vi "Default or Users Font.vi"(0 "PDF Report":refnum<class "PDF Report Class.lvclass">, 5 "Font":T1={"Name"="", "Size"=-1.0, "Color"=0, "Style"={"Bold"=FALSE, "Italic"=FALSE, "Underline"=FALSE, "Strikeout"=FALSE}, "Type"={"Type&direction"=enum."Select", "Embedded"=FALSE, "Encoding"=""}}, 11 "error in (no error)":errorcluster) -> (4 "PDF Report duplicate":refnum<class "PDF Report Class.lvclass">, 6 "Font OUT":T1={"Name"="Helvetica", "Size"=12.0, "Color"=0, "Style"={"Bold"=FALSE, "Italic"=FALSE, "Underline"=FALSE, "Strikeout"=FALSE}, "Type"={"Type&direction"=enum."Select", "Embedded"=FALSE, "Encoding"=""}}, 8 "Close Font Ref":bool=TRUE, 10 "Font Ref":refnum<k24>, 14 "Font Size":T2=18.0, 15 "error out":errorcluster)   [LabVIEW 2020, in "Exaprom PDF.lvlib" / "Font Class.lvclass"]
doc: "Version 1.0\nDeveloped by Jean-Marc Simard\nCopyright © 2012, Exaprom Inc.\nAll rights reserved.\nLicense: BSD\n\nWith iTextSharp 4.1.6 (http://itextsharp.sourceforge.net)\nunder Mozilla Public License Version 1.1\n(http://www.mozilla.org/MPL/MPL-1.1.html)"
uses:
  <userlib>/labview-PDF-writer-master/LV Class/Fonts Class/Font Class.lvclass
  <userlib>/labview-PDF-writer-master/LV Class/PDF Report Class/PDF Report Class.lvclass
  <userlib>/labview-PDF-writer-master/Controls/Font Controls/Font complete cluster.ctl
  <userlib>/labview-PDF-writer-master/Controls/Font Controls/Font size.ctl
  <userlib>/labview-PDF-writer-master/Controls/Font Controls/Font color.ctl
  <userlib>/labview-PDF-writer-master/Controls/Font Controls/Type and encoding.ctl
  <userlib>/labview-PDF-writer-master/Controls/Text Controls/Unicode/Type and run direction.ctl
  C:/Program Files (x86)/National Instruments/LabVIEW 2020/user.lib/labview-PDF-writer-master/DLL/itextsharp.dll
  DLL/itextsharp.dll
  <userlib>/labview-PDF-writer-master/Exaprom PDF.lvlib
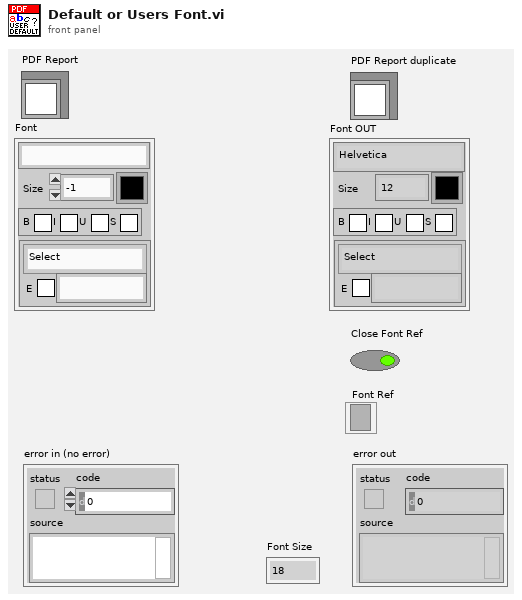
[diagram p1: front panel]
types:
  T1 = typedef "Exaprom PDF.lvlib/Font complete cluster.ctl" = cluster{"Name":string, "Size":T2, "Color":T3, "Style":cluster{"Bold":bool, "Italic":bool, "Underline":bool, "Strikeout":bool}, "Type":T4}
  T2 = typedef "Exaprom PDF.lvlib/Font size.ctl" = sgl
  T3 = typedef "Exaprom PDF.lvlib/Font color.ctl" = u32
  T4 = typedef "Exaprom PDF.lvlib/Type and encoding.ctl" = cluster{"Type&direction":T5, "Embedded":bool, "Encoding":string}
  T5 = typedef "Exaprom PDF.lvlib/Type and run direction.ctl" = enum16{"Select", "ASCII", "UTF-16", "UTF-16 (default)", "UTF-16 (LTR)", "UTF-16 (RTL)"}
  T6 = typedef "Exaprom PDF.lvlib/System Fonts.ctl" = cluster{"Font name [ ]":string[], "Font and file names [ ]":cluster{"Font name":string, "File name":string}[]}
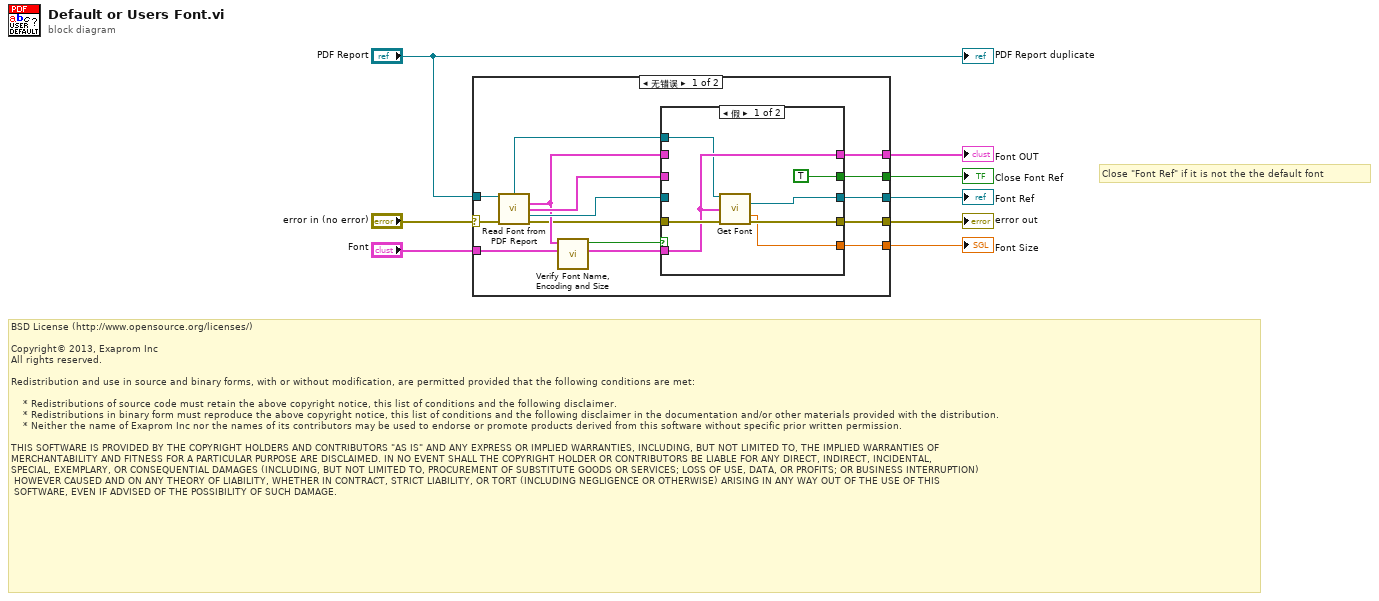
[diagram p0: block diagram]
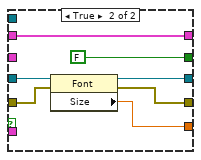
[diagram p2: hidden frame]
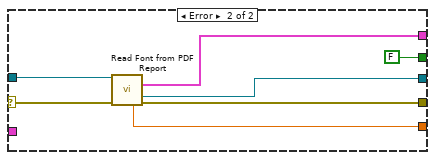
[diagram p3: hidden frame]
diagram:
  # "Close \"Font Ref\" if it is not the the default font"
  # "BSD License (http://www.opensource.org/licenses/)\n\nCopyright© 2013, Exaprom Inc\nAll rights reserved.\n\nRedistribution and use in source and binary forms, with or without modification, are permitted provided that the following conditions are met:\n\n    * Redistributions of source code must retain the above copyright notice, this list of conditions and the following disclaimer.\n    * Redistributions in binary form must reproduce the above copyright notice, this list of conditions and the following disclaimer in the documentation and/or other materials provided with the distribution.\n    * Neither the name of Exaprom Inc nor the names of its contributors may be used to endorse or promote products derived from this software without specific prior written permission.\n\nTHIS SOFTWARE IS PROVIDED BY THE COPYRIGHT HOLDERS AND CONTRIBUTORS \"AS IS\" AND ANY EXPRESS OR IMPLIED WARRANTIES, INCLUDING, BUT NOT LIMITED TO, THE IMPLIED WARRANTIES OF \nMERCHANTABILITY AND FITNESS FOR A PARTICULAR PURPOSE ARE DISCLAIMED. IN NO EVENT SHALL THE COPYRIGHT HOLDER OR CONTRIBUTORS BE LIABLE FOR ANY DIRECT, INDIRECT, INCIDENTAL,\nSPECIAL, EXEMPLARY, OR CONSEQUENTIAL DAMAGES (INCLUDING, BUT NOT LIMITED TO, PROCUREMENT OF SUBSTITUTE GOODS OR SERVICES; LOSS OF USE, DATA, OR PROFITS; OR BUSINESS INTERRUPTION)\n HOWEVER CAUSED AND ON ANY THEORY OF LIABILITY, WHETHER IN CONTRACT, STRICT LIABILITY, OR TORT (INCLUDING NEGLIGENCE OR OTHERWISE) ARISING IN ANY WAY OUT OF THE USE OF THIS\n SOFTWARE, EVEN IF ADVISED OF THE POSSIBILITY OF SUCH DAMAGE."
  n1 = case shown="无错误" "error in (no error)" {
    selector: "error in (no error)" -> [w9 w38]
    tunnel: [w23 w39] -> w8
    tunnel: [w22 w41] -> w7
    tunnel: [w21 FALSE] -> w6
    tunnel: [w20 w42] -> w5
    tunnel: "Font" -> [w19 _]
    tunnel: "PDF Report" -> [w15 w43]
    tunnel: [w16 w40] -> w2
    frame No Error {
      n2 = call <userlib>:"Read Font from PDF Report.vi"("PDF Report"=w15, "error in (no error)"=w9) -> ("Font Class.lvclass"=w11:refnum<class "Font Class.lvclass">, "Font OUT"=w12:T1, "System Fonts"=w14:T6, "Font Ref"=w13:refnum<k24>, "error out"=w10:errorcluster)  [unwired: 7 in, 2 out]
      n3 = call <userlib>:"Verify Font Name, Encoding and Size.vi"("Font IN"=w19, "Default Font cluster"=w12) -> ("Font OUT"=w17:T1, "Font = default font"=w18:bool)  [unwired: 8 in]
      n4 = case shown="假" w18 {
        tunnel: [w30 w36] -> w23
        tunnel: [w29 w37] -> w22
        tunnel: w10 -> [w28 w35]
        tunnel: [TRUE FALSE] -> w21
        tunnel: w13 -> [_ w33]
        tunnel: w17 -> [w26 _]
        tunnel: [w26 w32] -> w20
        tunnel: w12 -> [_ w32]
        tunnel: w14 -> [_ _]
        tunnel: [w25 w31] -> w16
        tunnel: w11 -> [w24 _]
        frame False {
          n5 = call <userlib>:"Get Font.vi"("Font"=w24, "Font IN"=w26, "error in (no error)"=w28) -> ("Font"=w29:refnum<k24>, "Font Size"=w25:T2, "error out"=w30:errorcluster)  [unwired: 8 in, 2 out]
        }
        frame True {
          n6 = property class="Font"(reference=w33, error in=w35) -> (reference out=w37:refnum<k24>, error out=w36:errorcluster, "Size"=w31:sgl)
        }
      }
    }
    frame Error {
      n7 = call <userlib>:"Read Font from PDF Report.vi"("PDF Report"=w43, "error in (no error)"=w38) -> ("Font OUT"=w42:T1, "Font Ref"=w41:refnum<k24>, "Font Size"=w40:T2, "error out"=w39:errorcluster)  [unwired: 7 in, 3 out]
    }
  }
  "error out" <- w8
  "Font Ref" <- w7
  "Font Size" <- w2
  "Close Font Ref" <- w6
  "Font OUT" <- w5
  "PDF Report duplicate" <- "PDF Report"
